vi "GPS Initialization Values.vi"(11 "VISA resource name":refnum<visa-resource-name>) -> (0 "error In":errorcluster, 2 "Buffer In":string="      ", 3 "VISA resource name In":refnum<visa-resource-name>)   [LabVIEW 2009]
uses:
  <vilib>/Instr/_visa.llb/VISA Configure Serial Port (Instr).vi
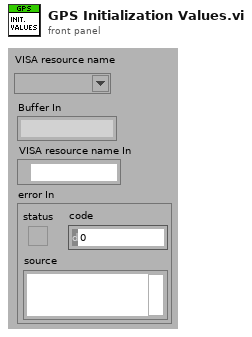
[diagram p1: front panel]
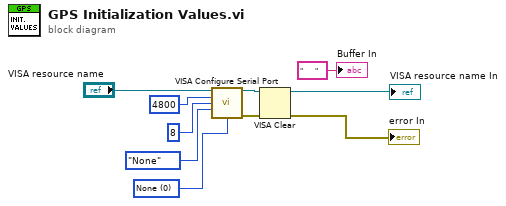
[diagram p0: block diagram]
diagram:
  w7 = u16 0 items=["None", "XON/XOFF", "RTS/CTS", "XON/XOFF & RTS/CTS", "DTR/DSR", "XON/XOFF & DTR/DSR"] ("flow control (0:none)")
  n1 = call-poly "VISA Configure Serial Port"("VISA resource name"="VISA resource name", "baud rate (9600)"=u32 4800, "data bits (8)"=u16 8, "parity (0:none)"=enum16{"None", "Odd", "Even", "Mark", "Space"}."None", "flow control (0:none)"=w7) -> ("VISA resource name out"=w5:refnum<visa-resource-name>, "error out"=w4:errorcluster)  [unwired: 9 in]
  n2 = VISA Clear(VISA resource name=w5, error in (no error)=w4) -> (VISA resource name out=→"VISA resource name In":refnum<visa-resource-name>, error out=→"error In":errorcluster)
  "Buffer In" <- "      " ("String")
